vi "2019-05-09_ForLoop.vi"() -> ()   [LabVIEW 2018]
panel:
  out "배열":u8[](array[numeric])
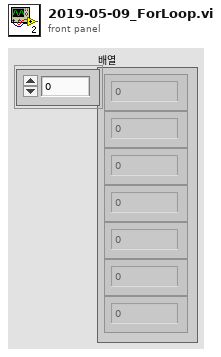
[diagram p1: front panel]
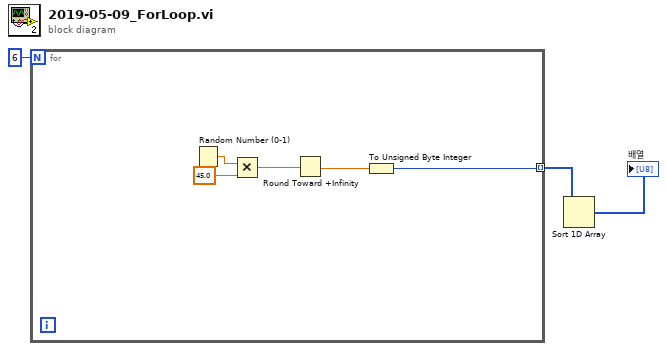
[diagram p0: block diagram]
diagram:
  n1 = for {
    N: 6 -> [_]
    tunnel: [w4] -> w2 mode=indexing
    n2 = Random Number (0-1)() -> (number: 0 to 1=w8:dbl)
    n3 = Multiply(x=w8, y=45.0) -> (x*y=w6:dbl)
    n4 = Round Toward +Infinity(x=w6) -> (ceil(x): smallest int >= x=w5:dbl)
    n5 = To Unsigned Byte Integer(number=w5) -> (unsigned 8bit integer=w4:u8)
  }
  n6 = Sort 1D Array(array=w2) -> (sorted array=→"배열":u8[])
